vi "File Process.vi"(10 "File Logging Process UE Refnum":T1, 11 "All Stop":refnum<user-event>) -> ()   [LabVIEW 2011]
doc: "Continuously generates File Logging and Error user events for the File Logging Process."
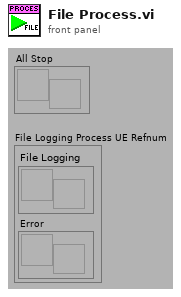
[diagram p1: front panel]
types:
  T1 = cluster{"File Logging":refnum<user-event>, "Error":refnum<user-event>}
  T2 = cluster{"seconds since 1Jan1904":timestamp, i32, "appended path":path}
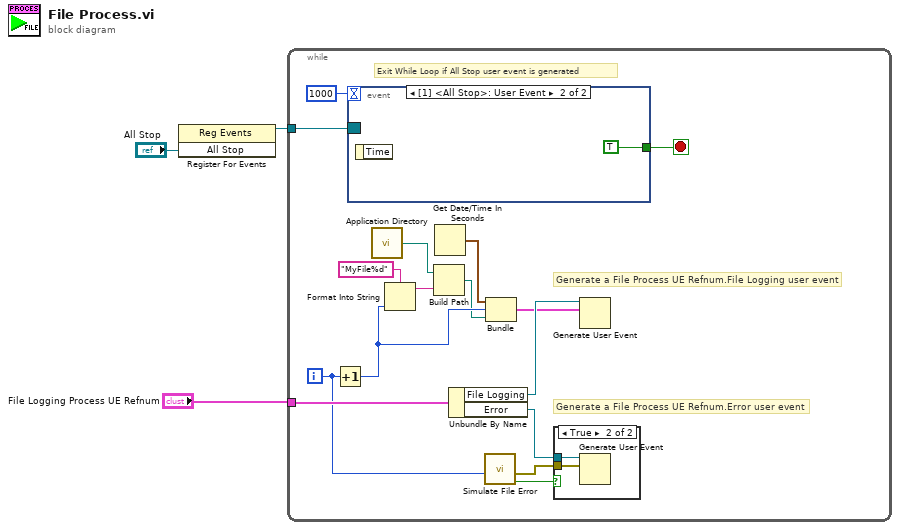
[diagram p0: block diagram]
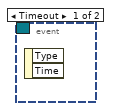
[diagram p3: hidden frame]
diagram:
  n1 = register-events("All Stop") -> (reference out=w2:refnum<event-registration>)  [unwired: 2 in, 1 out]
  n2 = while {
    tunnel: w2 -> [w17]
    tunnel: "File Logging Process UE Refnum" -> [w16]
    i -> [w15]
    stop <- w18 stop-if-true
    # "Generate a File Process UE Refnum.Error user event"
    # "Generate a File Process UE Refnum.File Logging user event"
    # "Exit While Loop if All Stop user event is generated"
    n3 = Increment(x=w15) -> (x+1=w9:i32)
    n4 = event shown="[1] <All Stop>: User Event" {
      selector: w17 -> [_ _]
      dyn-events: _ -> [_ _]
      timeout: 1000 -> [_ _]
      tunnel: [_ TRUE] -> w18
      event Timeout {
        n5 = event-data() -> ()  [unwired: 1 in, 2 out]
      }
      event User Event {
        n6 = event-data() -> ()  [unwired: 1 in, 1 out]
      }
    }
    n7 = call <vilib>:"Application Directory.vi"() -> ("Application Directory"=w6:path)
    n8 = Format Into String(format string="MyFile%d", w9) -> (resulting string=w5:string)  [unwired: 2 in, 1 out]
    n9 = Build Path(base path=w6, name or relative path=w5) -> (appended path=w4:path)
    n10 = Get Date/Time In Seconds() -> (seconds since 1Jan1904=w8:timestamp)
    n11 = Unbundle By Name(w16) -> ("File Logging"=w12:refnum<user-event>, "Error"=w13:refnum<user-event>)
    n12 = call "Simulate File Error.vi"("Iteration"=w15) -> ("Error?"=w11:bool, "error out"=w14:errorcluster)  [unwired: 9 in]
    n13 = Bundle("seconds since 1Jan1904"=w8, w9, "appended path"=w4) -> (w7:T2)  [unwired: 1 in]
    n14 = case shown="True" w11 {
      tunnel: w14 -> [_ w21]
      tunnel: w13 -> [_ w20]
      frame False {
      }
      frame True {
        n15 = Generate User Event(user event=w20, event data cluster=w21) -> ()  [unwired: 1 in, 2 out]
      }
    }
    n16 = Generate User Event(user event=w12, event data cluster=w7) -> ()  [unwired: 1 in, 2 out]
  }
